vi "控制板配置.vi"() -> ()   [LabVIEW 2010]
uses:
  全局量/全局_配置.vi
panel:
  in  "保存文件名":string
  in  "单选_LAN":bool
  in  "RS485_2端口":refnum<visa-resource-name>="COM1"
  in  "RS485_1端口":refnum<visa-resource-name>="COM1"
  in  "RS485波特率":T1(ring)
  in  "RS485路数":enum32{"0", "1", "2"}(ring)
  in  "R232端口":refnum<visa-resource-name>="COM1"
  in  "LAN端口":u32
  in  "str_IP":string
  in  "btn_返回":bool
  in  "RS232波特率":T1(ring)
  in  "RS232路数":enum32{"0", "1"}(ring)
  in  "AD输入幅值":enum32{"±3V", "±5V", "±12V"}(ring)
  in  "AD输入路数":T2(ring)
  in  "数字量输出路数":T2(ring)
  in  "CAN波特率":T3(ring)
  in  "CAN路数":string(combo)
  in  "DSP输入幅值":enum32{"±3V", "±5V", "±12V"}(ring)
  in  "DSP输入路数":T2(ring)
  in  "数字量输入路数":T2(ring)
  in  "btn_保存配置":bool
  in  "选择配置":T4(ring)
  # "控制板资源配置"
  # "数字量输出信号路数："
  # "数字量输入信号路数："
  # "外部AD模拟量输入信号路数："
  # "DSP模拟量输入信号路数："
  # "外部AD模拟量输入信号幅值："
  # "DSP模拟量输入信号幅值："
  # "RS232总线通信路数："
  # "RS485总线通信路数："
  # "1号"
  # "COM端口："
  # "COM端口："
  # "2号"
  # "RS232总线通信波特率："
  # "RS485总线通信波特率："
  # "控制板IP："
  # "CAN总线通信端口："
  # "控制板端口："
  # "CAN总线通信波特率："
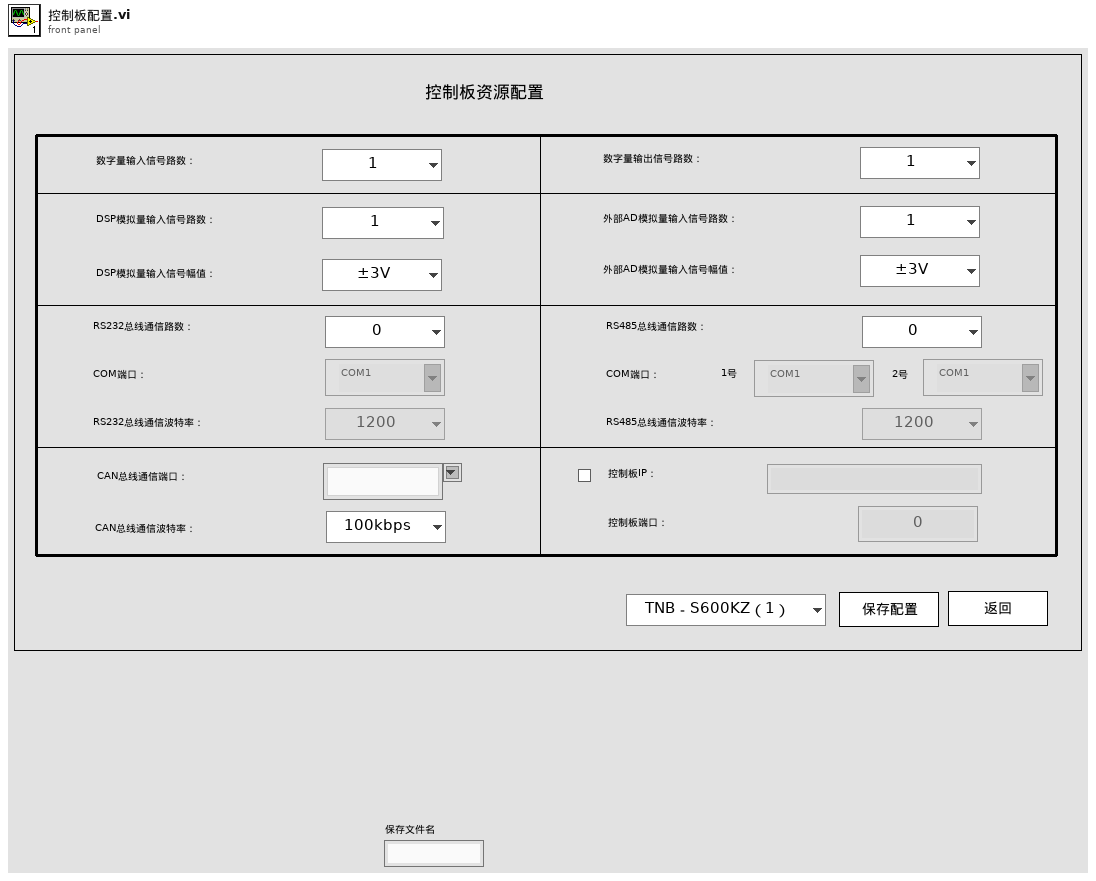
[diagram p1: front panel]
types:
  T1 = enum32{"1200", "2400", "4800", "9600", "19200", "57600", "115200", ""}
  T2 = enum32{"1", "2", "3", "4", "5", "6", "7", "8", "9", "10", "11", "12", "13", "14", "15", "16"}
  T3 = enum32{"100kbps", "200kbps", "250kbps", "500kbps", "1000kbps"}
  T4 = enum16{"TNB－S600KZ（1）", "TNB－S600KZ（2）", "TNB－S600KZ（3）", "TNB－S600KZ（4）", "TNB－S600KZ（5）"}
  T5 = enum8{"Enabled", "Disabled", "Disabled and Grayed Out"}
  T6 = cluster{"数字量输入信号路数":u32, "数字量输出信号路数":u32, "DSP模拟量输入信号路数":u32, "DSP模拟量输入信号幅值":u32, "AD模拟量输入信号路数":u32, "AD模拟量输入信号幅值":u32, "RS232端口":u32, "RS232通信路数":u32, "RS232波特率":u32, "RS485端口":u32, "RS485通信路数":u32, "RS485波特率":u32, "CAN通信端口":string, "CAN波特率":u32, "以太网选择?":bool, "控制板IP":string, "以太网端口":u32}
  T7 = cluster{"数字量输入路数":enum32{"1", "2", "3", "4", "5", "6", "7", "8", "9", "10", "11", "12", "13", "14", "15", "16"}, "数字量输出路数":enum32{"1", "2", "3", "4", "5", "6", "7", "8", "9", "10", "11", "12", "13", "14", "15", "16"}, "DSP输入路数":enum32{"1", "2", "3", "4", "5", "6", "7", "8", "9", "10", "11", "12", "13", "14", "15", "16"}, "DSP输入幅值":enum32{"±3V", "±5V", "±12V"}, "AD输入路数":enum32{"1", "2", "3", "4", "5", "6", "7", "8", "9", "10", "11", "12", "13", "14", "15", "16"}, "AD输入幅值":enum32{"±3V", "±5V", "±12V"}, "毫秒倍数":u32, "RS232路数":enum32{"0", "1"}, "RS232波特率":enum32{"1200", "2400", "4800", "9600", "19200", "57600", "115200", ""}, "毫秒倍数":u32, "RS485路数":enum32{"0", "1", "2"}, "RS485波特率":enum32{"1200", "2400", "4800", "9600", "19200", "57600", "115200", ""}, "CAN路数":string, "CAN波特率":enum32{"100kbps", "200kbps", "250kbps", "500kbps", "1000kbps"}, "单选_LAN":bool, "str_IP":string, "LAN端口":u32}
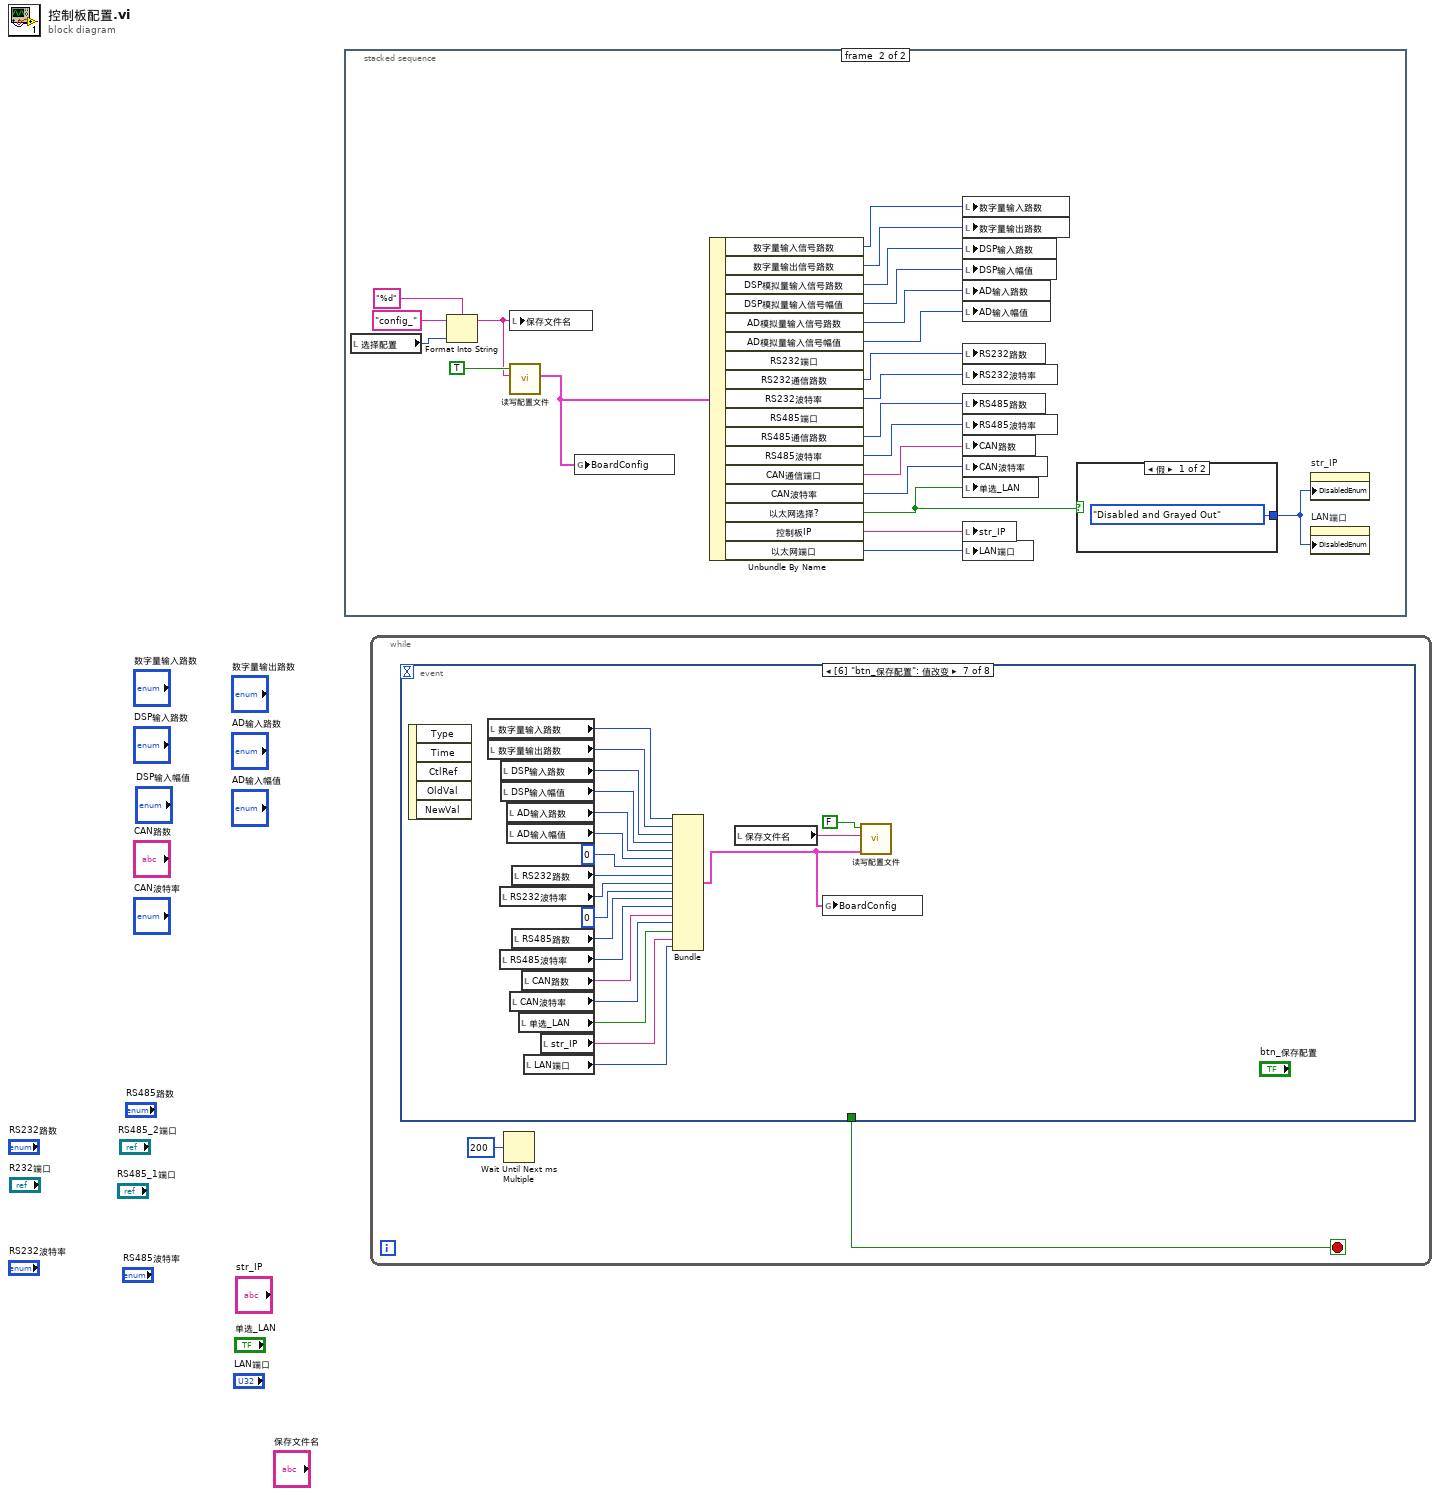
[diagram p0: block diagram]
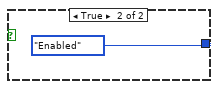
[diagram p3: hidden frame]
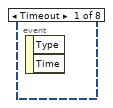
[diagram p4: hidden frame]
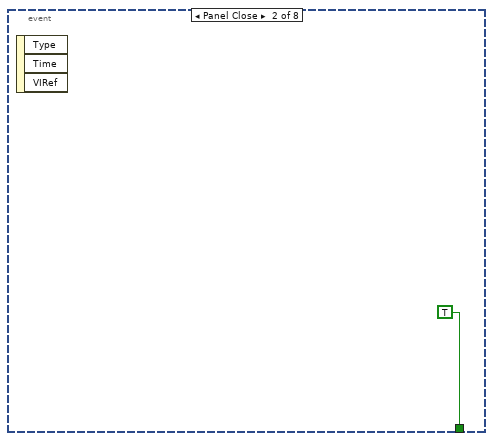
[diagram p5: hidden frame]
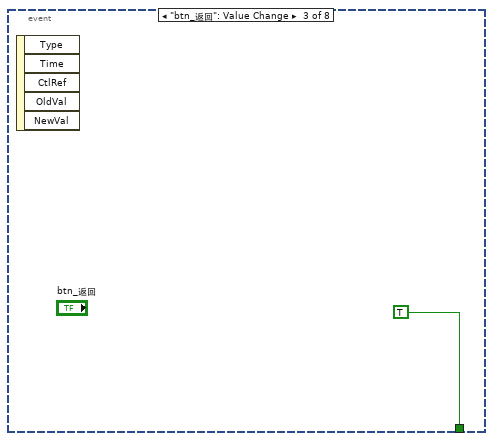
[diagram p6: hidden frame]
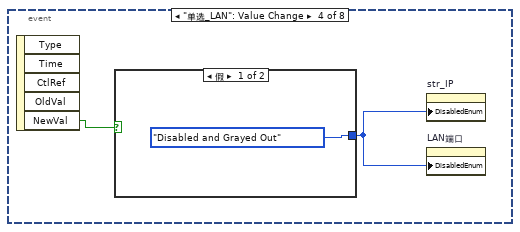
[diagram p7: hidden frame]
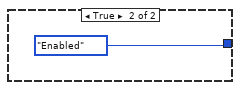
[diagram p8: hidden frame]
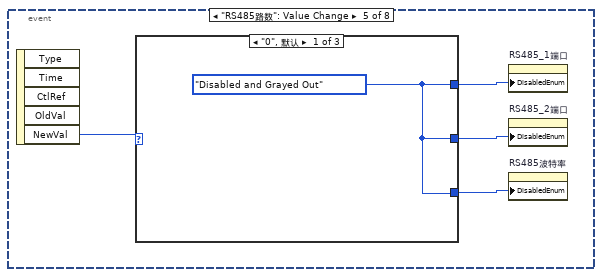
[diagram p9: hidden frame]
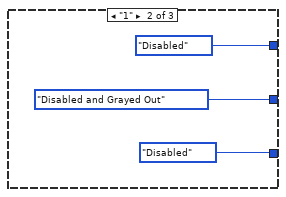
[diagram p10: hidden frame]
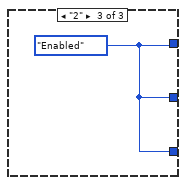
[diagram p11: hidden frame]
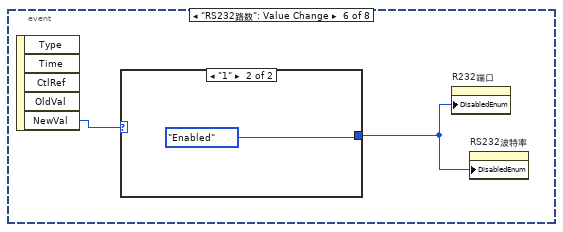
[diagram p12: hidden frame]
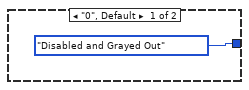
[diagram p13: hidden frame]
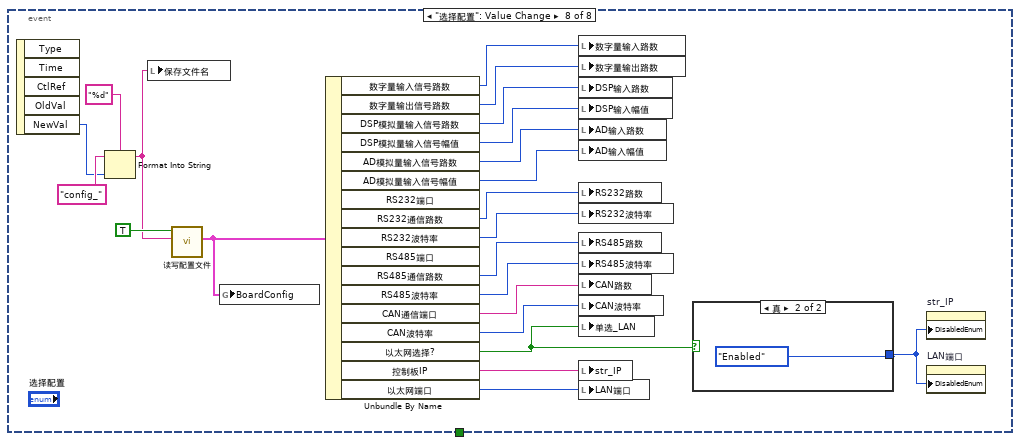
[diagram p14: hidden frame]
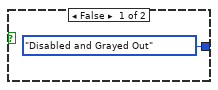
[diagram p15: hidden frame]
diagram:
  n1 = stacked-sequence {
    frame #0 {
    }
    frame #1 {
      n2 = local read "选择配置"() -> (w4:T4)
      n3 = Format Into String(format string="%d", initial string="config_", w4) -> (resulting string=w2:string)  [unwired: 1 in, 1 out]
      n4 = local write "保存文件名"(w2) -> ()
      n5 = call "读写配置文件.vi"("文件名称"=w2, "m_bRead"=TRUE) -> ("BoardConfig_output"=w1:T6)  [unwired: 9 in]
      n6 = global write "全局_配置.vi" "BoardConfig"(w1) -> ()
      n7 = Unbundle By Name(w1) -> ("数字量输入信号路数"=w7:u32, "数字量输出信号路数"=w8:u32, "DSP模拟量输入信号路数"=w9:u32, "DSP模拟量输入信号幅值"=w10:u32, "AD模拟量输入信号路数"=w11:u32, "AD模拟量输入信号幅值"=w12:u32, "RS232通信路数"=w13:u32, "RS232波特率"=w14:u32, "RS485通信路数"=w15:u32, "RS485波特率"=w16:u32, "CAN通信端口"=w17:string, "CAN波特率"=w18:u32, "以太网选择?"=w22:bool, "控制板IP"=w19:string, "以太网端口"=w20:u32)  [unwired: 2 out]
      n8 = local write "数字量输入路数"(w7) -> ()
      n9 = local write "数字量输出路数"(w8) -> ()
      n10 = local write "DSP输入路数"(w9) -> ()
      n11 = local write "DSP输入幅值"(w10) -> ()
      n12 = local write "AD输入路数"(w11) -> ()
      n13 = local write "AD输入幅值"(w12) -> ()
      n14 = local write "RS232路数"(w13) -> ()
      n15 = local write "RS232波特率"(w14) -> ()
      n16 = local write "RS485路数"(w15) -> ()
      n17 = local write "RS485波特率"(w16) -> ()
      n18 = local write "CAN路数"(w17) -> ()
      n19 = local write "CAN波特率"(w18) -> ()
      n20 = local write "单选_LAN"(w22) -> ()
      n21 = local write "str_IP"(w19) -> ()
      n22 = local write "LAN端口"(w20) -> ()
      n23 = case shown="假" w22 {
        tunnel: [T5."Disabled and Grayed Out" ("禁用") T5."Enabled" ("禁用")] -> w21
        frame False {
        }
        frame True {
        }
      }
      n24 = property on="str_IP" class="Str"("DisabledEnum"=w21) -> ()  [unwired: 2 in, 2 out]
      n25 = property on="LAN端口" class="DigNum (严格)"("DisabledEnum"=w21) -> ()  [unwired: 2 in, 2 out]
    }
  }
  n26 = while {
    stop <- w26 stop-if-true
    n27 = event shown="[6] \"btn_保存配置\": 值改变" {
      selector: _ -> [_ _ _ _ _ _ _ _]
      dyn-events: _ -> [_ _ _ _ _ _ _ _]
      timeout: _ -> [_ _ _ _ _ _ _ _]
      tunnel: [_ TRUE TRUE _ _ _ _ _] -> w26
      event Timeout {
        n28 = event-data() -> ()  [unwired: 1 in, 2 out]
      }
      event Panel Close {
        n29 = event-data() -> ()  [unwired: 1 in, 3 out]
      }
      event "btn_返回": Value Change {
        n30 = event-data() -> ()  [unwired: 1 in, 5 out]
      }
      event "单选_LAN": Value Change {
        n31 = event-data() -> ("NewVal"=w30:bool)  [unwired: 1 in, 4 out]
        n32 = case shown="假" w30 {
          tunnel: [T5."Disabled and Grayed Out" ("禁用") T5."Enabled" ("禁用")] -> w29
          frame False {
          }
          frame True {
          }
        }
        n33 = property on="str_IP" class="Str"("DisabledEnum"=w29) -> ()  [unwired: 2 in, 2 out]
        n34 = property on="LAN端口" class="DigNum (严格)"("DisabledEnum"=w29) -> ()  [unwired: 2 in, 2 out]
      }
      event "RS485路数": Value Change {
        n35 = event-data() -> ("NewVal"=w36:enum32{"0", "1", "2"})  [unwired: 1 in, 4 out]
        n36 = case shown="\"0\", 默认" w36 {
          tunnel: [w37 T5."Disabled" ("禁用") w41] -> w35
          tunnel: [w37 T5."Disabled" ("禁用") w41] -> w34
          tunnel: [w37 T5."Disabled and Grayed Out" ("禁用") w41] -> w33
          frame "0", Default {
            w37 = T5."Disabled and Grayed Out" ("禁用")
          }
          frame "1" {
          }
          frame "2" {
            w41 = T5."Enabled" ("禁用")
          }
        }
        n37 = property on="RS485_1端口" class="VISAName"("DisabledEnum"=w35) -> ()  [unwired: 2 in, 2 out]
        n38 = property on="RS485_2端口" class="VISAName"("DisabledEnum"=w33) -> ()  [unwired: 2 in, 2 out]
        n39 = property on="RS485波特率" class="Enum (严格)"("DisabledEnum"=w34) -> ()  [unwired: 2 in, 2 out]
      }
      event "RS232路数": Value Change {
        n40 = event-data() -> ("NewVal"=w43:enum32{"0", "1"})  [unwired: 1 in, 4 out]
        n41 = case shown="\"1\"" w43 {
          tunnel: [T5."Disabled and Grayed Out" ("禁用") T5."Enabled" ("禁用")] -> w42
          frame "0", Default {
          }
          frame "1" {
          }
        }
        n42 = property on="R232端口" class="VISAName"("DisabledEnum"=w42) -> ()  [unwired: 2 in, 2 out]
        n43 = property on="RS232波特率" class="Enum (严格)"("DisabledEnum"=w42) -> ()  [unwired: 2 in, 2 out]
      }
      event "btn_保存配置": Value Change {
        n44 = event-data() -> ()  [unwired: 1 in, 5 out]
        n45 = local read "数字量输入路数"() -> (w63:T2)
        n46 = local read "数字量输出路数"() -> (w62:T2)
        n47 = local read "RS232波特率"() -> (w55:T1)
        n48 = local read "RS485波特率"() -> (w52:T1)
        n49 = local read "DSP输入路数"() -> (w61:T2)
        n50 = local read "DSP输入幅值"() -> (w60:enum32{"±3V", "±5V", "±12V"})
        n51 = local read "AD输入路数"() -> (w59:T2)
        n52 = local read "AD输入幅值"() -> (w58:enum32{"±3V", "±5V", "±12V"})
        n53 = local read "CAN波特率"() -> (w50:T3)
        n54 = local read "RS232路数"() -> (w56:enum32{"0", "1"})
        n55 = local read "RS485路数"() -> (w53:enum32{"0", "1", "2"})
        n56 = local read "单选_LAN"() -> (w49:bool)
        n57 = local read "CAN路数"() -> (w51:string)
        n58 = local read "LAN端口"() -> (w47:u32)
        n59 = local read "str_IP"() -> (w48:string)
        n60 = Bundle("数字量输入路数"=w63, "数字量输出路数"=w62, "DSP输入路数"=w61, "DSP输入幅值"=w60, "AD输入路数"=w59, "AD输入幅值"=w58, "毫秒倍数"=u32 0, "RS232路数"=w56, "RS232波特率"=w55, "毫秒倍数"=u32 0, "RS485路数"=w53, "RS485波特率"=w52, "CAN路数"=w51, "CAN波特率"=w50, "单选_LAN"=w49, "str_IP"=w48, "LAN端口"=w47) -> (w46:T7)  [unwired: 1 in]
        n61 = local read "保存文件名"() -> (w64:string)
        n62 = global write "全局_配置.vi" "BoardConfig"(w46) -> ()
        n63 = call "读写配置文件.vi"("BoardConfig_input"=w46, "文件名称"=w64, "m_bRead"=FALSE) -> ()  [unwired: 8 in, 1 out]
      }
      event "选择配置": Value Change {
        n64 = event-data() -> ("NewVal"=w85:T4)  [unwired: 1 in, 4 out]
        n65 = Format Into String(format string="%d", initial string="config_", w85) -> (resulting string=w83:string)  [unwired: 1 in, 1 out]
        n66 = local write "保存文件名"(w83) -> ()
        n67 = call "读写配置文件.vi"("文件名称"=w83, "m_bRead"=TRUE) -> ("BoardConfig_output"=w66:T6)  [unwired: 9 in]
        n68 = global write "全局_配置.vi" "BoardConfig"(w66) -> ()
        n69 = Unbundle By Name(w66) -> ("数字量输入信号路数"=w82:u32, "数字量输出信号路数"=w81:u32, "DSP模拟量输入信号路数"=w80:u32, "DSP模拟量输入信号幅值"=w79:u32, "AD模拟量输入信号路数"=w78:u32, "AD模拟量输入信号幅值"=w77:u32, "RS232通信路数"=w76:u32, "RS232波特率"=w75:u32, "RS485通信路数"=w74:u32, "RS485波特率"=w73:u32, "CAN通信端口"=w72:string, "CAN波特率"=w71:u32, "以太网选择?"=w67:bool, "控制板IP"=w70:string, "以太网端口"=w69:u32)  [unwired: 2 out]
        n70 = local write "数字量输入路数"(w82) -> ()
        n71 = local write "数字量输出路数"(w81) -> ()
        n72 = local write "DSP输入路数"(w80) -> ()
        n73 = local write "DSP输入幅值"(w79) -> ()
        n74 = local write "AD输入路数"(w78) -> ()
        n75 = local write "AD输入幅值"(w77) -> ()
        n76 = local write "RS232路数"(w76) -> ()
        n77 = local write "RS232波特率"(w75) -> ()
        n78 = local write "RS485路数"(w74) -> ()
        n79 = local write "RS485波特率"(w73) -> ()
        n80 = local write "CAN路数"(w72) -> ()
        n81 = local write "CAN波特率"(w71) -> ()
        n82 = local write "单选_LAN"(w67) -> ()
        n83 = local write "str_IP"(w70) -> ()
        n84 = local write "LAN端口"(w69) -> ()
        n85 = case shown="真" w67 {
          tunnel: [T5."Disabled and Grayed Out" ("禁用") T5."Enabled" ("禁用")] -> w68
          frame False {
          }
          frame True {
          }
        }
        n86 = property on="str_IP" class="Str"("DisabledEnum"=w68) -> ()  [unwired: 2 in, 2 out]
        n87 = property on="LAN端口" class="DigNum (严格)"("DisabledEnum"=w68) -> ()  [unwired: 2 in, 2 out]
      }
    }
    n88 = Wait Until Next ms Multiple(millisecond multiple=u32 200 ("毫秒倍数")) -> ()  [unwired: 1 out]
  }
